vi "Configure GPIO.vi"(5 "Purpose (\"GPIO\")":string="GPIO", 7 "GPIO #":T3=-1, 8 "error in (no error)":errorcluster, 9 "GPIO Pull (None)":T2, 10 "GPIO Direction":T1, 11 "Session in":refnum<class "Session.lvclass">) -> (0 "error out":errorcluster, 3 "Session out":refnum<class "Session.lvclass">)   [LabVIEW 2020, in "CTI.lvlib" / "Session.lvclass"]
uses:
  Session.lvclass
  GPIO Number.ctl
  GPIO Pull.ctl
  GPIO Direction.ctl
  Session.lvclass/Session.ctl
  71948ec3-9283-445f-8a06-496401628b65.vi
  Is Full Errors.vi
  Check Errors.vi
  CTI.lvlib
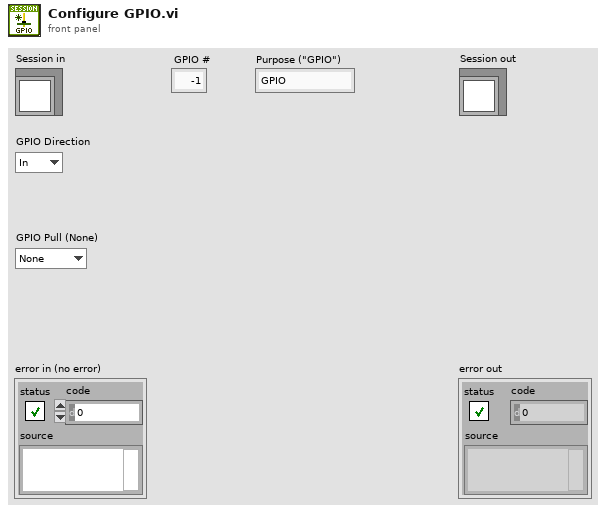
[diagram p1: front panel]
types:
  T1 = typedef "CTI.lvlib/GPIO Direction.ctl" = enum16{"In", "Out"}
  T2 = typedef "CTI.lvlib/GPIO Pull.ctl" = enum16{"None", "Up", "Down", "Both"}
  T3 = typedef "CTI.lvlib/GPIO Number.ctl" = i8
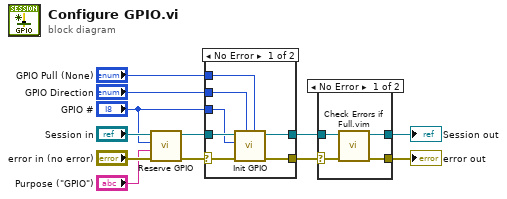
[diagram p0: block diagram]
diagram:
  n1 = call "Reserve GPIO.vi"("error in (no error)"="error in (no error)", "Purpose"="Purpose (\"GPIO\")", "GPIO #"="GPIO #", "Session in"="Session in") -> ("error out"=w7:errorcluster, "Session out"=w6:refnum<class "Session.lvclass">)  [unwired: 6 in]
  n2 = case shown="No Error" w7 {
    selector: w7 -> [w19 w21]
    tunnel: w6 -> [w18 w20]
    tunnel: [w17 w20] -> w5
    tunnel: [w16 w21] -> w4
    tunnel: "GPIO Direction" -> [w15 _]
    tunnel: "GPIO Pull (None)" -> [w14 _]
    tunnel: "GPIO #" -> [w13 _]
    frame No Error {
      n3 = call-dynamic "Init GPIO.vi"("GPIO Pull (None)"=w14, "GPIO Direction"=w15, "error in (no error)"=w19, "GPIO #"=w13, "Session in"=w18) -> ("error out"=w16:errorcluster, "Session out"=w17:refnum<class "Session.lvclass">)  [unwired: 5 in]
    }
    frame Error {
    }
  }
  n4 = case shown="No Error" w4 {
    selector: w4 -> [w22 w26]
    tunnel: w5 -> [w23 w27]
    tunnel: [w24 w27] -> w9
    tunnel: [w25 w26] -> w8
    frame No Error {
      n5 = call "Check Errors if Full.vim"("error in (no error)"=w22, "Session in"=w23) -> ("error out"=w25:errorcluster, "Session out"=w24:refnum<class "Session.lvclass">)  [unwired: 8 in]
    }
    frame Error {
    }
  }
  "error out" <- w8
  "Session out" <- w9
